vi "Create File Response.vi"(8 "error in (no error)":errorcluster, 10 "Content-Type (Auto)":string, 11 "Path":path) -> (0 "error out":errorcluster, 3 "File Response out":refnum<class "File Response.lvclass">)   [LabVIEW 2020, in "HTTP Utils.lvlib" / "File Response.lvclass"]
uses:
  File Response.lvclass
  File Response.lvclass/File Response.ctl
  Response/Response.lvclass
  HTTP Utils.lvlib
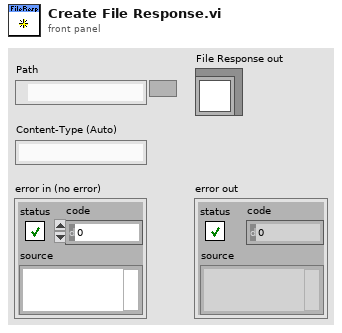
[diagram p1: front panel]
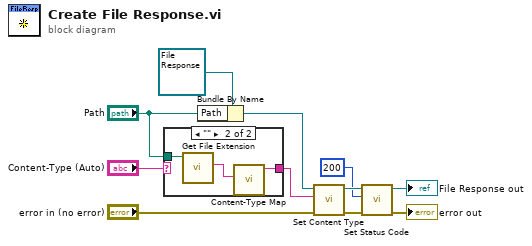
[diagram p0: block diagram]
diagram:
  n1 = case shown="\"\"" "Content-Type (Auto)" {
    selector: "Content-Type (Auto)" -> [w12 _]
    tunnel: "Path" -> [_ w15]
    tunnel: [w12 w13] -> w1
    frame Default {
    }
    frame "" {
      n2 = call <vilib>:"Get File Extension.vi"("file"=w15) -> ("lowercase file extension"=w14:string)  [unwired: 6 in, 4 out]
      n3 = call "Content-Type Map.vi"("File Extension"=w14) -> ("Extension Content-Type"=w13:string)  [unwired: 9 in, 1 out]
    }
  }
  n4 = Bundle By Name(cluster=refnum<class "File Response.lvclass"> refnum ("File Response in"), "Path"="Path") -> (w2:refnum<class "File Response.lvclass">)
  n5 = call "Set Content Type.vi"("error in (no error)"="error in (no error)", "Content-Type"=w1, "Response in"=w2) -> ("error out"=w5:errorcluster, "Response out"=w4:refnum<class "File Response.lvclass">)  [unwired: 7 in]
  n6 = call "Set Status Code.vi"("error in (no error)"=w5, "Status Code"=u16 200, "Response in"=w4) -> ("error out"=→"error out":errorcluster, "Response out"=→"File Response out":refnum<class "File Response.lvclass">)  [unwired: 7 in]
